vi "XML Script - SubVI (Path).vi"(0 "x":i32=-1, 1 "y":i32=-1, 2 "out":i32=-1, 3 "IgnoreSearchDialogIfVIMissing?":bool, 4 "path":path, 6 "name":string, 9 "prefix (name)":string, 10 "in":i32=-1) -> (5 "name (wire source)":string, 7 "XML Script Command - SubVI":string)   [LabVIEW 2020]
panel:
  # "position"
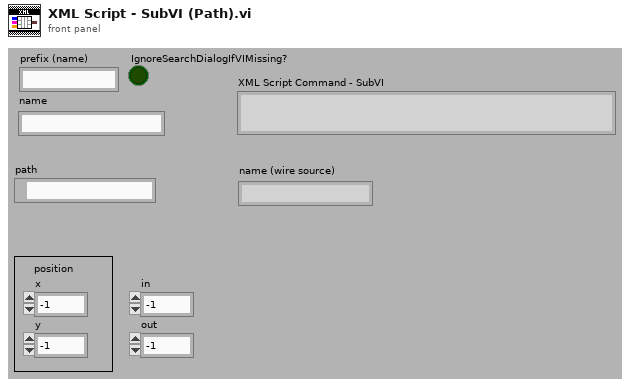
[diagram p1: front panel]
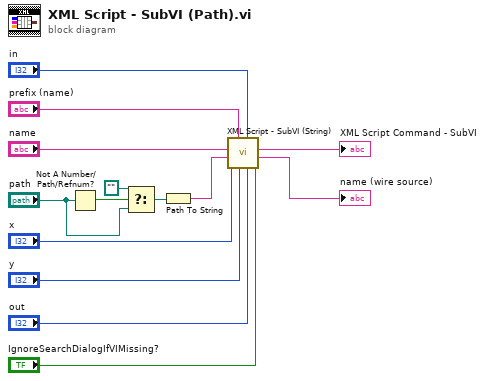
[diagram p0: block diagram]
diagram:
  n1 = Not A Number/Path/Refnum?(number/path/refnum="path") -> (NaN/Path/Refnum?=w5:bool)
  n2 = Select(t=path "", s=w5, f="path") -> (s? t:f=w3:path)
  n3 = Path To String(path=w3) -> (string=w2:string)
  n4 = call <vilib>:"XML Script - SubVI (String).vi"("x"="x", "y"="y", "out"="out", "IgnoreSearchDialogIfVIMissing?"="IgnoreSearchDialogIfVIMissing?", "path"=w2, "name"="name", "prefix (name)"="prefix (name)", "in"="in") -> ("name (wire source)"=→"name (wire source)":string, "XML Script Command - SubVI"=→"XML Script Command - SubVI":string)  [unwired: 2 in]
